vi "Get Descendant Libraries.vi"(11 "error in":errorcluster) -> (4 "project out":refnum<vi>, 6 "all descendents":refnum<vi>[](array[refnum]), 15 "error out":errorcluster)   [LabVIEW 2021, in "Converter.lvlib"]
uses:
  Converter.lvlib
  Converter Reusables/Converter Reusables.lvlib
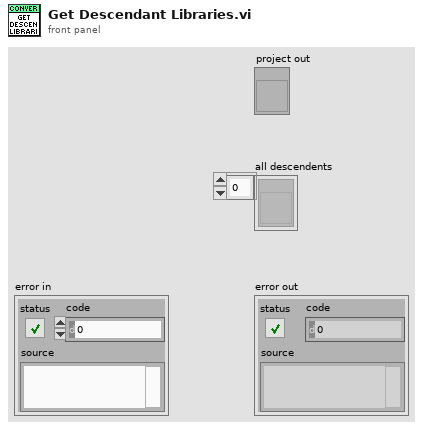
[diagram p1: front panel]
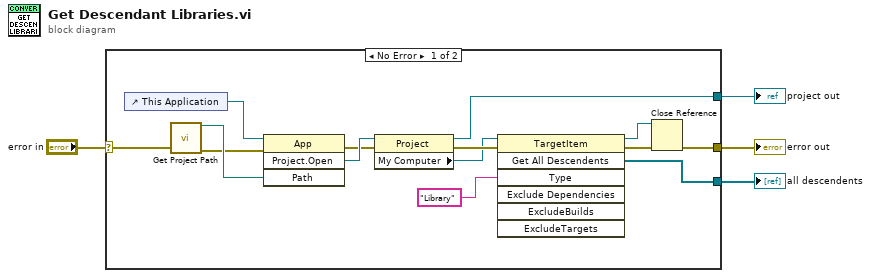
[diagram p0: block diagram]
diagram:
  n1 = case shown="No Error" "error in" {
    selector: "error in" -> [w15 w19]
    tunnel: [w17 w19] -> w4
    tunnel: [w13 _] -> w2
    tunnel: [w5 _] -> w1
    frame No Error {
      n2 = control-ref of="This Application"() -> (w6:refnum<vi>)
      n3 = call "Get Project Path.vi"("error in"=w15) -> ("project path out"=w18:path, "error out"=w16:errorcluster)  [unwired: 13 in]
      n4 = invoke class="App" method="Project.Open"(reference=w6, error in=w16, "Path"=w18) -> (error out=w7:errorcluster, "Project:Open"=w14:refnum<vi>)  [unwired: 1 in, 2 out]
      n5 = property class="Project"(reference=w14, error in=w7) -> (reference out=w5:refnum<vi>, error out=w12:errorcluster, "My Computer"=w8:refnum<vi>)
      n6 = invoke class="TargetItem" method="Get All Descendents"(reference=w8, error in=w12, "Type"="Library") -> (reference out=w11:refnum<vi>, error out=w10:errorcluster, "All Descendents"=w13:refnum<vi>[])  [unwired: 4 in, 4 out]
      n7 = Close Reference(reference=w11, error in (no error)=w10) -> (error out=w17:errorcluster)
    }
    frame Error {
    }
  }
  "error out" <- w4
  "project out" <- w1
  "all descendents" <- w2
